vi "Move Tilt Stage.vi"(2 "Axis Control (DO NOT USE)":T4={"A"=0.0, "A'"=0.0, "B"=6.0, "B'"=6.0, "C"=4, "Run A?"=FALSE, "Run B?"=FALSE, "Run C?"=FALSE, "Run A'?"=FALSE, "Run B'?"=FALSE}, 3 "Advanced Control":T5={"X"=0, "theta Y"=0.0, "Y"=6.0, "theta Z"=6.0, "Z"=4.0, "Run X?"=FALSE, "Run Y?"=FALSE, "Run Z?"=FALSE, "Run theta Y?"=FALSE, "Run theta Z?"=FALSE}) -> (0 "Axis Positions":T2, 1 "Advanced Positions":T3)   [LabVIEW 2016]
uses:
  C:/Users/UsphereLab/Documents/GitHub/Optlev/LabView Code/Examples/Tilt Stage/CmdLib.dll
  Examples/Tilt Stage/CmdLib.dll
panel:
  in  "Axis inputs 5":T1={"Relative Steps"=0, "Motor Number"=1, "Run?"=FALSE, "Filename"=path "position.lvm", "CmdLib In"=refnum, "Device Address In"=0, "DeviceKey In"=""}
  in  "Axis inputs 4":T1={"Relative Steps"=0, "Motor Number"=1, "Run?"=FALSE, "Filename"=path "position.lvm", "CmdLib In"=refnum, "Device Address In"=0, "DeviceKey In"=""}
  in  "Axis inputs 3":T1={"Relative Steps"=0, "Motor Number"=1, "Run?"=FALSE, "Filename"=path "position.lvm", "CmdLib In"=refnum, "Device Address In"=0, "DeviceKey In"=""}
  in  "B Inputs":T1={"Relative Steps"=0, "Motor Number"=1, "Run?"=FALSE, "Filename"=path "position.lvm", "CmdLib In"=refnum, "Device Address In"=0, "DeviceKey In"=""}
  in  "A inputs":T1={"Relative Steps"=0, "Motor Number"=1, "Run?"=FALSE, "Filename"=path "position.lvm", "CmdLib In"=refnum, "Device Address In"=0, "DeviceKey In"=""}
  in  "Axis Positions 2":T2
  in  "Advanced Positions 2":T3
  out "Position error out":errorcluster
  in  "stop":bool
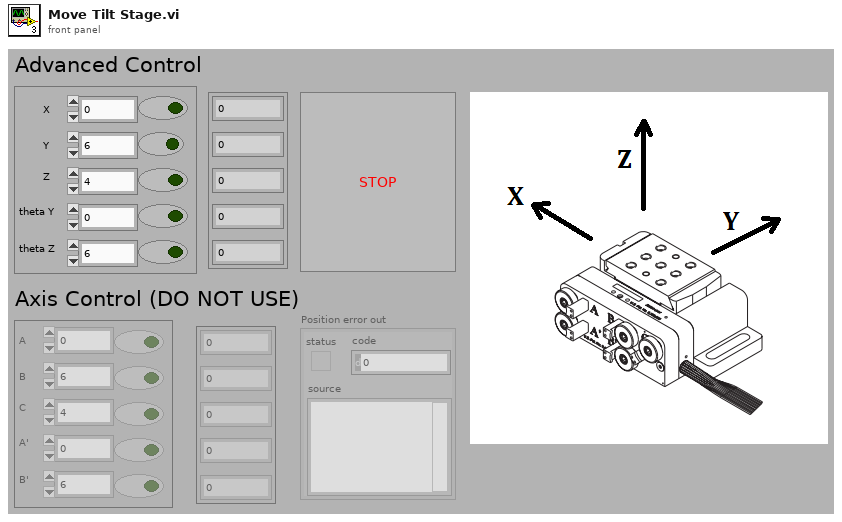
[diagram p1: front panel]
types:
  T1 = cluster{"Relative Steps":i32, "Motor Number":i32, "Run?":bool, "Filename":path, "CmdLib In":refnum<k24>, "Device Address In":i32, "DeviceKey In":string}
  T2 = cluster{"Position of A":i32, "Position of B":i32, "Position of C":i32, "Position of A'":i32, "Position of B'":i32}
  T3 = cluster{"X position":i32, "Y position":i32, "Z position":i32, "theta Y position":i32, "theta Z position":i32}
  T4 = cluster{"A":dbl, "A'":dbl, "B":dbl, "B'":dbl, "C":i32, "Run A?":bool, "Run B?":bool, "Run C?":bool, "Run A'?":bool, "Run B'?":bool}
  T5 = cluster{"X":i32, "theta Y":dbl, "Y":dbl, "theta Z":dbl, "Z":dbl, "Run X?":bool, "Run Y?":bool, "Run Z?":bool, "Run theta Y?":bool, "Run theta Z?":bool}
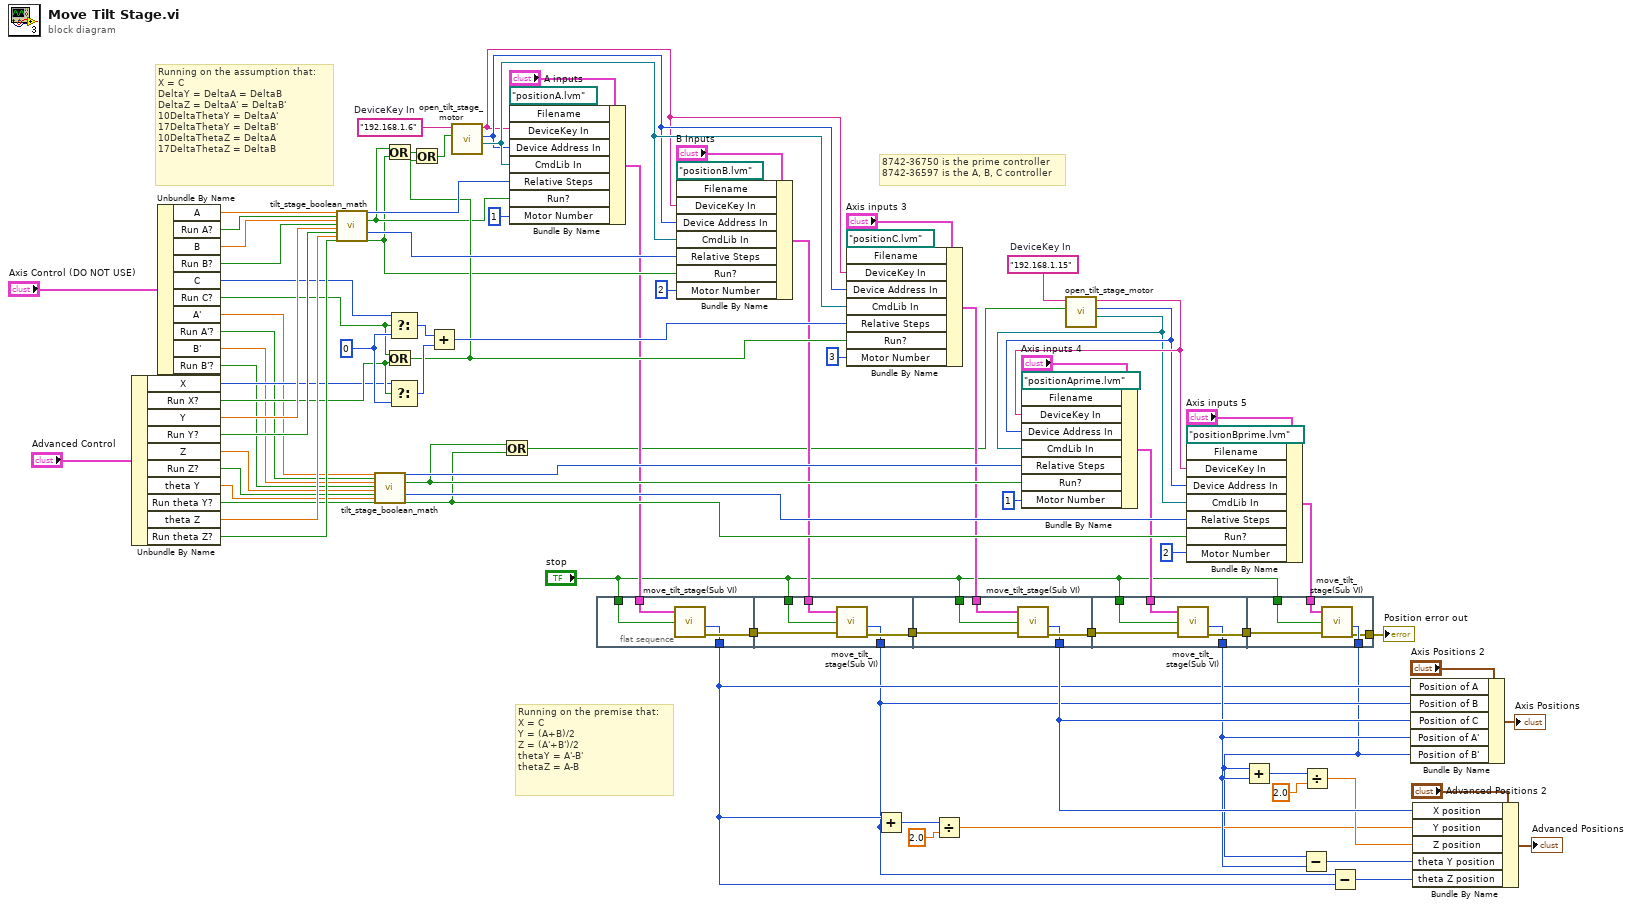
[diagram p0: block diagram]
diagram:
  w89 = 0 ("f")
  w49 = "192.168.1.15"  # DeviceKey In
  w59 = "192.168.1.6"  # DeviceKey In
  # "Running on the premise that:\nX = C\nY = (A+B)/2\nZ = (A'+B')/2\nthetaY = A'-B'\nthetaZ = A-B"
  # "Running on the assumption that:\nX = C\nDeltaY = DeltaA = DeltaB\nDeltaZ = DeltaA' = DeltaB'\n10DeltaThetaY = DeltaA'\n17DeltaThetaY = DeltaB'\n10DeltaThetaZ = DeltaA\n17DeltaThetaZ = DeltaB"
  # "8742-36750 is the prime controller\n8742-36597 is the A, B, C controller"
  n1 = Unbundle By Name("Advanced Control") -> ("X"=w69:i32, "Run X?"=w70:bool, "Y"=w76:dbl, "Run Y?"=w75:bool, "Z"=w64:dbl, "Run Z?"=w63:bool, "theta Y"=w62:dbl, "Run theta Y?"=w61:bool, "theta Z"=w74:dbl, "Run theta Z?"=w73:bool)
  n2 = Unbundle By Name("Axis Control (DO NOT USE)") -> ("A"=w80:dbl, "Run A?"=w79:bool, "B"=w78:dbl, "Run B?"=w77:bool, "C"=w72:i32, "Run C?"=w71:bool, "A'"=w68:dbl, "Run A'?"=w67:bool, "B'"=w66:dbl, "Run B'?"=w65:bool)
  n3 = call "tilt_stage_boolean_math.vi"("A"=w80, "Run A?"=w79, "B"=w78, "Run B?"=w77, "Y/Z"=w76, "Run Y/Z?"=w75, "theta"=w74, "Run theta?"=w73) -> ("A"=w53:i32, "A?"=w42:bool, "B"=w51:i32, "B?"=w41:bool)  [unwired: 16 in]
  n4 = call "tilt_stage_boolean_math.vi"("A"=w68, "Run A?"=w67, "B"=w66, "Run B?"=w65, "Y/Z"=w64, "Run Y/Z?"=w63, "theta"=w62, "Run theta?"=w61) -> ("A"=w40:i32, "A?"=w39:bool, "B"=w30:i32, "B?"=w29:bool)  [unwired: 16 in]
  n5 = Or(x=w42, y=w41) -> (x .or. y?=w44:bool)
  n6 = Or(x=w71, y=w70) -> (x .or. y?=w43:bool)
  n7 = Select(t=w72, s=w71, f=w89) -> (s? t:f=w88:i32)
  n8 = Select(t=w69, s=w70, f=w89) -> (s? t:f=w87:i32)
  n9 = Or(x=w44, y=w43) -> (x .or. y?=w3:bool)
  n10 = Add(x=w88, y=w87) -> (x+y=w50:i32)
  n11 = call "open_tilt_stage_motor.vi"("Open device?"=w3, "DeviceKey In"=w59) -> ("CmdLib Out"=w56:refnum<k24>, "Device Address"=w55:i32, "DeviceKey Out"=w54:string)  [unwired: 2 in, 1 out]
  n12 = Or(x=w39, y=w29) -> (x .or. y?=w2:bool)
  n13 = Bundle By Name(cluster="A inputs", "Filename"=path "positionA.lvm", "DeviceKey In"=w54, "Device Address In"=w55, "CmdLib In"=w56, "Relative Steps"=w53, "Run?"=w42, "Motor Number"=1) -> (w28:T1)
  n14 = flat-sequence {
    tunnel: "stop" -> [w93]
    tunnel: w28 -> [w92]
    tunnel: [w91] -> w22
    tunnel: [w90] -> w8
    tunnel: w27 -> [w98]
    tunnel: "stop" -> [w97]
    tunnel: w22 -> [w96]
    tunnel: [w95] -> w21
    tunnel: [w94] -> w7
    tunnel: w26 -> [w103]
    tunnel: "stop" -> [w102]
    tunnel: w21 -> [w101]
    tunnel: [w100] -> w20
    tunnel: [w99] -> w17
    tunnel: w24 -> [w108]
    tunnel: "stop" -> [w107]
    tunnel: w20 -> [w106]
    tunnel: [w105] -> w19
    tunnel: [w104] -> w9
    tunnel: [w110] -> w5
    tunnel: w19 -> [w111]
    tunnel: "stop" -> [w112]
    tunnel: w25 -> [w113]
    tunnel: [w109] -> w1
    frame #0 {
      n15 = call "move_tilt_stage(Sub VI).vi"("Axis inputs"=w92, "stop"=w93) -> ("Position Status"=w90:i32, "error out"=w91:errorcluster)  [unwired: 1 in, 2 out]
    }
    frame #1 {
      n16 = call "move_tilt_stage(Sub VI).vi"("Axis inputs"=w98, "stop"=w97, "error in (no error)"=w96) -> ("Position Status"=w94:i32, "error out"=w95:errorcluster)  [unwired: 2 out]
    }
    frame #2 {
      n17 = call "move_tilt_stage(Sub VI).vi"("Axis inputs"=w103, "stop"=w102, "error in (no error)"=w101) -> ("Position Status"=w99:i32, "error out"=w100:errorcluster)  [unwired: 2 out]
    }
    frame #3 {
      n18 = call "move_tilt_stage(Sub VI).vi"("Axis inputs"=w108, "stop"=w107, "error in (no error)"=w106) -> ("Position Status"=w104:i32, "error out"=w105:errorcluster)  [unwired: 2 out]
    }
    frame #4 {
      n19 = call "move_tilt_stage(Sub VI).vi"("Axis inputs"=w113, "stop"=w112, "error in (no error)"=w111) -> ("Position Status"=w110:i32, "error out"=w109:errorcluster)  [unwired: 2 out]
    }
  }
  n20 = Bundle By Name(cluster="B Inputs", "Filename"=path "positionB.lvm", "DeviceKey In"=w54, "Device Address In"=w55, "CmdLib In"=w56, "Relative Steps"=w51, "Run?"=w41, "Motor Number"=2) -> (w27:T1)
  n21 = Bundle By Name(cluster="Axis inputs 3", "Filename"=path "positionC.lvm", "DeviceKey In"=w54, "Device Address In"=w55, "CmdLib In"=w56, "Relative Steps"=w50, "Run?"=w43, "Motor Number"=3) -> (w26:T1)
  n22 = Add(x=w8, y=w7) -> (x+y=w16:i32)
  n23 = Divide(x=w16, y=2.0) -> (x/y=w6:dbl)
  n24 = call "open_tilt_stage_motor.vi"("Open device?"=w2, "DeviceKey In"=w49) -> ("CmdLib Out"=w33:refnum<k24>, "Device Address"=w34:i32, "DeviceKey Out"=w35:string)  [unwired: 2 in, 1 out]
  n25 = Bundle By Name(cluster="Axis inputs 4", "Filename"=path "positionAprime.lvm", "DeviceKey In"=w35, "Device Address In"=w34, "CmdLib In"=w33, "Relative Steps"=w40, "Run?"=w39, "Motor Number"=1) -> (w24:T1)
  n26 = Bundle By Name(cluster="Axis inputs 5", "Filename"=path "positionBprime.lvm", "DeviceKey In"=w35, "Device Address In"=w34, "CmdLib In"=w33, "Relative Steps"=w30, "Run?"=w29, "Motor Number"=2) -> (w25:T1)
  n27 = Add(x=w5, y=w9) -> (x+y=w14:i32)
  n28 = Subtract(x=w5, y=w9) -> (x-y=w11:i32)
  n29 = Divide(x=w14, y=2.0) -> (x/y=w10:dbl)
  n30 = Subtract(x=w7, y=w8) -> (x-y=w12:i32)
  n31 = Bundle By Name(cluster="Axis Positions 2", "Position of A"=w8, "Position of B"=w7, "Position of C"=w17, "Position of A'"=w9, "Position of B'"=w5) -> (→"Axis Positions":T2)
  n32 = Bundle By Name(cluster="Advanced Positions 2", "X position"=w17, "Y position"=w6, "Z position"=w10, "theta Y position"=w11, "theta Z position"=w12) -> (→"Advanced Positions":T3)
  "Position error out" <- w1
